vi "Read StandardBroadcasts.vi"(8 "error in (no error)":errorcluster, 11 "JQMHCore in":refnum<class "RQMHModule.lvclass">) -> (0 "error out":errorcluster, 2 "Broadcasts":T1, 3 "JQMHCore out":refnum<class "RQMHModule.lvclass">)   [LabVIEW 2024, in "RQMHModule.lvclass"]
uses:
  RQMHModule.lvclass
  StandardBroadcasts.ctl
  Shared/Died.ctl
  Started.ctl
  RQMHModule.lvclass/RQMHModule.ctl
  Shared/RQMHShared.lvlib
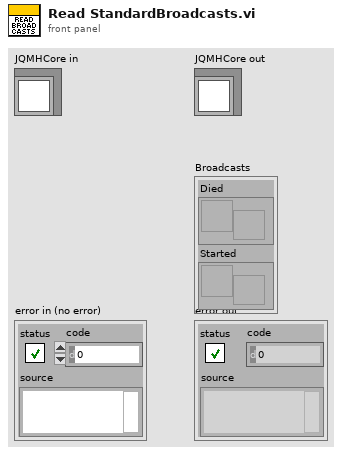
[diagram p1: front panel]
types:
  T1 = typedef "RQMHModule.lvclass/StandardBroadcasts.ctl" = cluster{"Died":refnum<user-event>, "Started":refnum<user-event>}
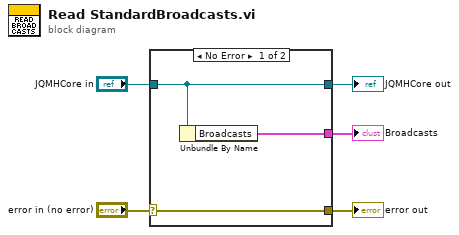
[diagram p0: block diagram]
diagram:
  n1 = case shown="No Error" "error in (no error)" {
    selector: "error in (no error)" -> [w8 w9]
    tunnel: [w8 w9] -> w4
    tunnel: [w7 w10] -> w2
    tunnel: "JQMHCore in" -> [w7 w10]
    tunnel: [w6 _] -> w1
    frame No Error {
      n2 = Unbundle By Name(w7) -> ("Broadcasts"=w6:T1)
    }
    frame Error {
    }
  }
  "error out" <- w4
  "JQMHCore out" <- w2
  "Broadcasts" <- w1
